vi "Module Loop.vi"(8 "error in (no error)":errorcluster, 11 "ValveSimModule in":refnum<class "ValveSimModule.lvclass">) -> (0 "error out":errorcluster, 3 "ValveSimModule out":refnum<class "ValveSimModule.lvclass">)   [LabVIEW 2023, in "VolatusScratch.lvlib" / "ValveSimModule.lvclass"]
uses:
  ValveSimModule.lvclass
  ValveSimModule.lvclass/ValveSimModule.ctl
  Volatus/Module/Module.lvclass
  lv-vecto/Vecto/Group DBL/Group DBL.lvclass
  lv-vecto/Vecto/Vecto.lvlib
  lv-vecto/Vecto/Channel DBL/Channel DBL.lvclass
  C:/dev/volatus/mts-volatus-super/libs/lv-volatus/Volatus/Module/Module.lvclass
  C:/dev/volatus/mts-volatus-super/libs/lv-volatus/VolatusScratch/ValveSimModule/ValveSimModule.lvclass
  C:/dev/volatus/mts-volatus-super/libs/lv-vecto/Vecto/Group/Group.lvclass
  C:/dev/volatus/mts-volatus-super/libs/lv-vecto/Vecto/Group DBL/Group DBL.lvclass
  Valve State.ctl
panel:
  in  "Both Limits":bool
  out "State":T1
  in  "Skip Publish":bool
  out "Energized":bool
  out "Open":bool
  out "Closed":bool
  out "Command":bool
  in  "Energize Delay":dbl=0.3
  in  "Close Time":dbl=0.8
  in  "Open Time":dbl=0.6
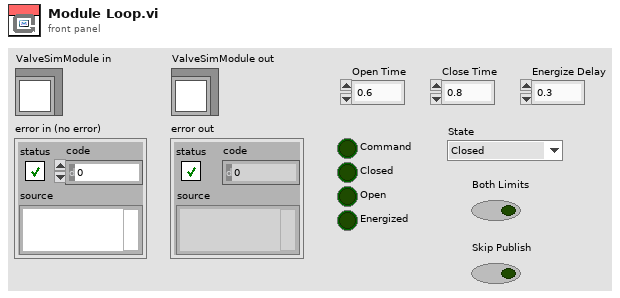
[diagram p1: front panel]
types:
  T1 = typedef "VolatusScratch.lvlib/ValveSimModule.lvclass/Valve State.ctl" = enum16{"Closed", "Energize", "Open", "Opened", "Deenergize", "Close"}
  T2 = cluster{"Open Time":dbl, "Close Time":dbl, "Energize Delay":dbl}
  T3 = typedef "CmdDigitalMultiple.lvlib/Data.ctl" = cluster{"values":T4[]}
  T4 = typedef "CmdDigital.lvlib/Data.ctl" = cluster{"channel":string, "value":bool}
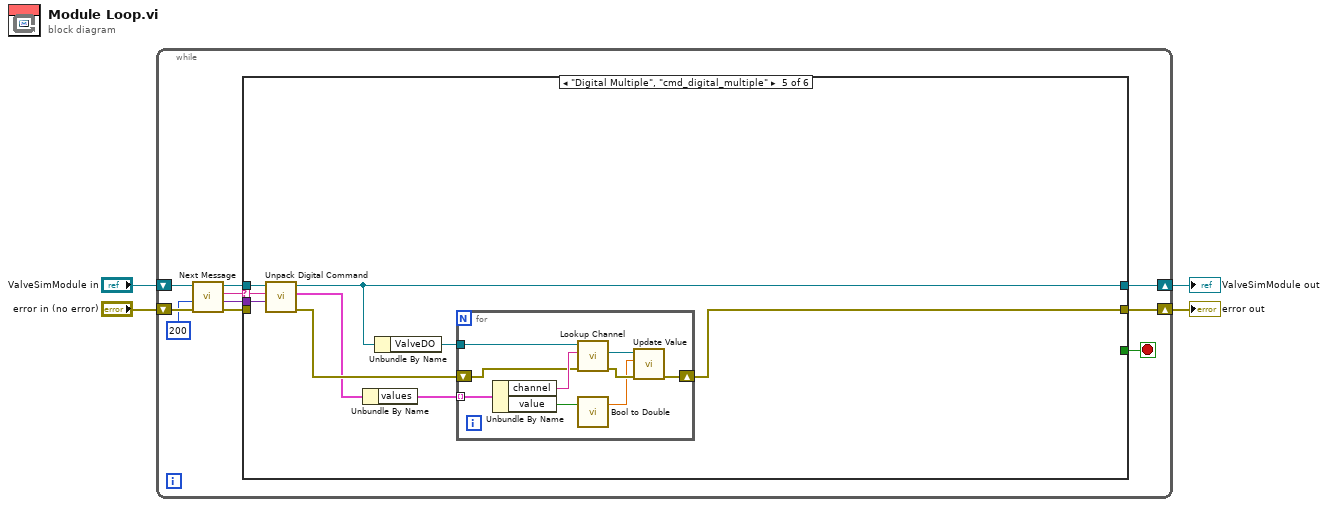
[diagram p0: block diagram]
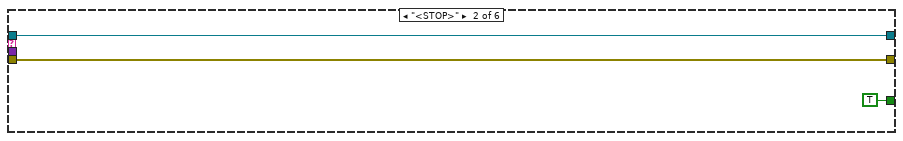
[diagram p3: hidden frame]
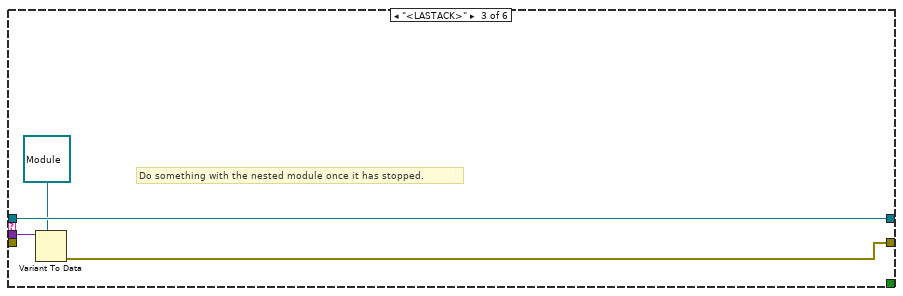
[diagram p4: hidden frame]
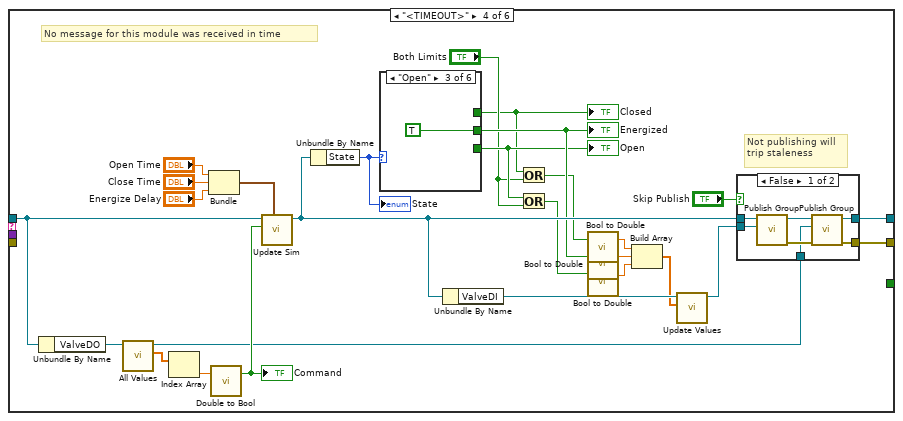
[diagram p5: hidden frame]
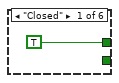
[diagram p7: hidden frame]
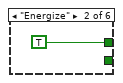
[diagram p8: hidden frame]
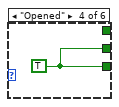
[diagram p9: hidden frame]
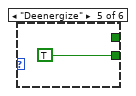
[diagram p10: hidden frame]
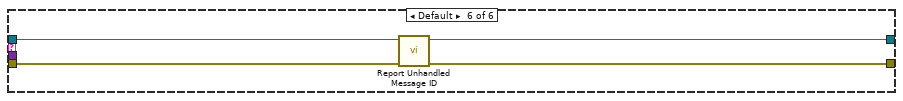
[diagram p12: hidden frame]
diagram:
  n1 = while {
    shift-right: [w9] -> w2
    shift-left: "ValveSimModule in" -> [w14]
    shift-right: [w8] -> w1
    shift-left: "error in (no error)" -> [w13]
    stop <- w7 stop-if-true
    n2 = call "Next Message.vi"("error in (no error)"=w13, "Timeout/Period ms (-1)"=200 ("Timeout ms (-1)"), "Module in"=w14) -> ("error out"=w12:errorcluster, "Data"=w6:variant, "ID"=w11:string, "Module out"=w10:refnum<class "ValveSimModule.lvclass">)  [unwired: 5 in]
    n3 = case shown="\"Digital Multiple\", \"cmd_digital_multiple\"" w11 {
      selector: w11 -> [_ _ _ _ w67 _]
      tunnel: w12 -> [w15 w18 _ _ _ w85]
      tunnel: w10 -> [w16 w19 w23 w50 w69 w83]
      tunnel: [w16 w19 w23 w33 w64 w82] -> w9
      tunnel: [w15 w18 w20 w31 w70 w84] -> w8
      tunnel: [_ TRUE _ _ _ _] -> w7
      tunnel: w6 -> [_ _ w22 _ w68 _]
      frame "<CLOSE>" {
      }
      frame "<STOP>" {
      }
      frame "<LASTACK>" {
        # "Do something with the nested module once it has stopped."
        n4 = Variant To Data(type=refnum<class "Module.lvclass"> refnum ("Volatus:Module"), Variant=w22) -> (error out=w20:errorcluster)  [unwired: 1 in, 1 out]
      }
      frame "<TIMEOUT>" {
        # "Not publishing will trip staleness"
        # "No message for this module was received in time"
        n5 = Unbundle By Name(w50) -> ("ValveDO"=w49:refnum<class "Group DBL.lvclass">)
        n6 = call "All Values.vi"("Group in"=w49) -> ("Scaled"=w48:dbl[], "Group out"=w32:refnum<class "Group DBL.lvclass">)  [unwired: 6 in, 3 out]
        n7 = Index Array(array=w48) -> (element=w47:dbl)  [unwired: 1 in]
        n8 = Bundle("Open Time"="Open Time", "Close Time"="Close Time", "Energize Delay"="Energize Delay") -> (w42:T2)  [unwired: 1 in]
        n9 = call "Double to Bool.vi"("Double"=w47) -> ("Bool"=w46:bool)  [unwired: 2 in]
        "Command" <- w46
        n10 = call "Update Sim.vi"("Timings"=w42, "Command"=w46, "ValveSimModule in"=w50) -> ("ValveSimModule out"=w40:refnum<class "ValveSimModule.lvclass">)  [unwired: 7 in, 1 out]
        n11 = Unbundle By Name(w40) -> ("State"=w41:T1)
        "State" <- w41
        n12 = case shown="\"Open\"" w41 {
          tunnel: [TRUE TRUE _ _ _ _] -> w25
          tunnel: [_ _ TRUE w62 _ _] -> w29
          tunnel: [_ _ _ w62 TRUE _] -> w28
          frame "Closed" {
          }
          frame "Energize" {
          }
          frame "Open" {
          }
          frame "Opened" {
            w62 = TRUE
          }
          frame "Deenergize" {
          }
          frame "Close" {
          }
        }
        "Closed" <- w25
        "Open" <- w28
        "Energized" <- w29
        n13 = Unbundle By Name(w40) -> ("ValveDI"=w36:refnum<class "Group DBL.lvclass">)
        n14 = Or(x=w25, y="Both Limits") -> (x .or. y?=w24:bool)
        n15 = Or(x=w28, y="Both Limits") -> (x .or. y?=w27:bool)
        n16 = call "Bool to Double.vi"("Bool"=w24) -> ("Double"=w39:dbl)  [unwired: 2 in]
        n17 = call "Bool to Double.vi"("Bool"=w29) -> ("Double"=w38:dbl)  [unwired: 2 in]
        n18 = call "Bool to Double.vi"("Bool"=w27) -> ("Double"=w37:dbl)  [unwired: 2 in]
        n19 = Build Array(w39, w38, w37) -> (w35:dbl[])
        n20 = call "Update Values.vi"("Values"=w35, "Group in"=w36) -> ("Group out"=w34:refnum<class "Group DBL.lvclass">)  [unwired: 8 in, 1 out]
        n21 = case shown="False" "Skip Publish" {
          tunnel: w40 -> [w56 w58]
          tunnel: w34 -> [w54 _]
          tunnel: [w53 w58] -> w33
          tunnel: w32 -> [w52 _]
          tunnel: [w51 _] -> w31
          frame False {
            n22 = call "Publish Group.vi"("Group"=w54, "Module in"=w56) -> ("error out"=w57:errorcluster, "Module out"=w55:refnum<class "ValveSimModule.lvclass">)  [unwired: 8 in]
            n23 = call "Publish Group.vi"("error in (no error)"=w57, "Group"=w52, "Module in"=w55) -> ("error out"=w51:errorcluster, "Module out"=w53:refnum<class "ValveSimModule.lvclass">)  [unwired: 7 in]
          }
          frame True {
          }
        }
      }
      frame "Digital Multiple", "cmd_digital_multiple" {
        n24 = call "Unpack Digital Command.vi"("Data"=w68, "Type"=w67, "Module in"=w69) -> ("error out"=w72:errorcluster, "CmdDigitalMultiple"=w66:T3, "Module out"=w64:refnum<class "ValveSimModule.lvclass">)  [unwired: 4 in, 2 out]
        n25 = Unbundle By Name(w66) -> ("values"=w65:T4[])
        n26 = Unbundle By Name(w64) -> ("ValveDO"=w71:refnum<class "Group DBL.lvclass">)
        n27 = for {
          tunnel: w71 -> [w81]
          tunnel: w65 -> [w74] mode=indexing
          shift-right: [w75] -> w70
          shift-left: w72 -> [w73]
          n28 = Unbundle By Name(w74) -> ("channel"=w80:string, "value"=w78:bool)
          n29 = call "Lookup Channel.vi"("error in (no error)"=w73, "Channel Name"=w80, "Group in"=w81) -> ("error out"=w77:errorcluster, "Channel"=w79:refnum<class "Channel DBL.lvclass">)  [unwired: 6 in, 1 out]
          n30 = call "Bool to Double.vi"("Bool"=w78) -> ("Double"=w76:dbl)  [unwired: 2 in]
          n31 = call "Update Value.vi"("error in (no error)"=w77, "Value"=w76, "Channel in"=w79) -> ("error out"=w75:errorcluster)  [unwired: 7 in, 1 out]
        }
      }
      frame Default {
        n32 = call "Report Unhandled Message ID.vi"("error in (no error)"=w85, "Module in"=w83) -> ("error out"=w84:errorcluster, "Module out"=w82:refnum<class "ValveSimModule.lvclass">)  [unwired: 8 in]
      }
    }
  }
  "error out" <- w1
  "ValveSimModule out" <- w2
